vi "String2ArrayDouble.vi"(2 "R_message 1":string) -> (0 "Array":sgl[](array[numeric]))   [LabVIEW 2022 SP3]
panel:
  out "subarray":u8[](array[numeric]) format="%x"
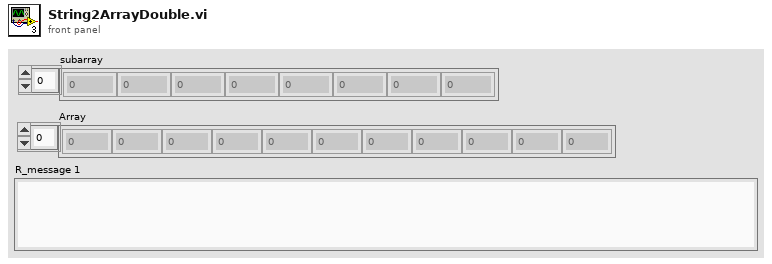
[diagram p1: front panel]
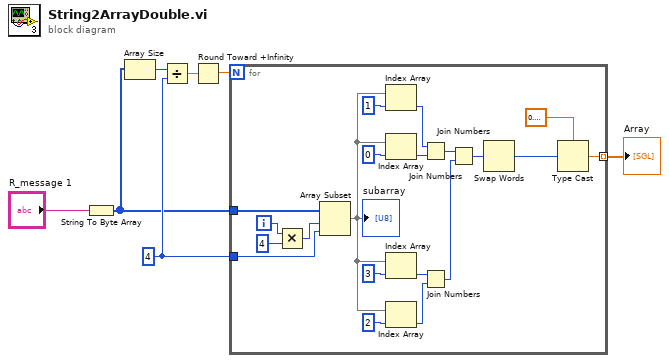
[diagram p0: block diagram]
diagram:
  w5 = 4 ("length")
  n1 = String To Byte Array(string="R_message 1") -> (unsigned byte array=w2:u8[])
  n2 = Array Size(array=w2) -> (size(s)=w6:i32)
  n3 = Divide(x=w6, y=w5) -> (x/y=w4:dbl)
  n4 = Round Toward +Infinity(x=w4) -> (ceil(x): smallest int >= x=w3:dbl)
  n5 = for {
    N: w3 -> [_]
    tunnel: w2 -> [w27]
    tunnel: w5 -> [w26]
    tunnel: [w24] -> w1 mode=indexing
    i -> [w10]
    n6 = Multiply(x=w10, y=4) -> (x*y=w8:i32)
    n7 = Array Subset(array=w27, index=w8, length=w26) -> (w15:u8[])
    "subarray" <- w15
    n8 = Index Array(array=w15, index=1) -> (element=w17:u8)
    n9 = Index Array(array=w15, index=0) -> (element=w16:u8)
    n10 = Index Array(array=w15, index=3) -> (element=w14:u8)
    n11 = Index Array(array=w15, index=2) -> (element=w13:u8)
    n12 = Join Numbers(hi=w17, lo=w16) -> ((hi.lo)=w18:u16)
    n13 = Join Numbers(hi=w14, lo=w13) -> ((hi.lo)=w19:u16)
    n14 = Join Numbers(hi=w18, lo=w19) -> ((hi.lo)=w12:u32)
    n15 = Swap Words(1:w12) -> (0:w11:u32)
    n16 = Type Cast(type=sgl 0.1, x=w11) -> (*(type *) &x=w24:sgl)
  }
  "Array" <- w1
